vi "IandQ_Dat_ACQ.vi"() -> ()   [LabVIEW 2022 SP3]
doc: "I. Description:\nThis example demonstrates how to acquire a continuous amount of data (Waveform) using the DAQ device's internal clock.\n\nII. Instructions for Running:\n1. Create an analog input voltage channel.\n2. Set the rate for the sample clock. Additionally, define the sample mode to be continuous.\n3. Call the Start VI to start the acquisition.\n4. Read the waveform data in a loop until the user hits the stop button or an error occurs.\nNote: This example reads data from one or more channels and returns an array of data. Use the Index Array function to access an individual channel of data.\n5. Call the Clear Task VI to clear the Task.\n6. Use the popup dialog box to display an error if any.\n\nIV. I/O Connections Overview:\nMake sure your signal input terminal matches the Physical Channel I/O Control. For further connection information, refer to your hardware reference manual."
uses:
  <vilib>/Utility/error.llb/DialogType.ctl
  <vilib>/DAQmx/read.llb/DAQmx Read (Analog Wfm 1Chan NSamp).vi
  <vilib>/DAQmx/create/channels.llb/DAQmx Create Channel (AI-Voltage-Basic).vi
  <vilib>/DAQmx/configure/timing.llb/DAQmx Timing (Sample Clock).vi
  <vilib>/DAQmx/miscellaneous.llb/DAQmx Fill In Error Info.vi
panel:
  in  "Samples to Read":i32=1000
  in  "Physical Channel":tag="Dev1/ai0"
  in  "Minimum Value":dbl=-10.0 format="%0.2f"
  in  "Maximum Value":dbl=10.0 format="%0.2f"
  in  "stop":bool
  in  "Sample Rate":dbl=10000.0 caption="Sample Rate (Hz)" format="%0.2f"
  out "Measurement":waveform(dbl)(graph)
  # "For instructions, select Help>>Show Context Help"
  # "Channel Parameters"
  # "Timing Parameters"
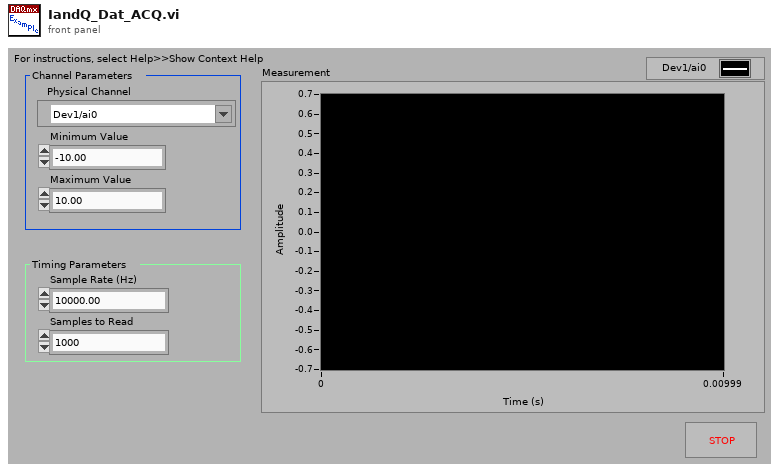
[diagram p1: front panel]
types:
  T1 = typedef "DialogType.ctl" = u16
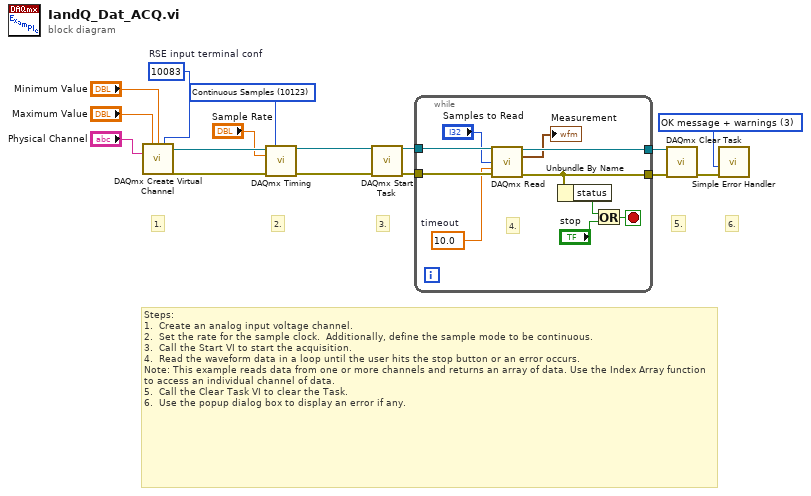
[diagram p0: block diagram]
diagram:
  w1 = 10083  # RSE input terminal conf
  w2 = T1 3 items=["no dialog", "OK message", "continue or stop message", "OK message + warnings", "continue/stop + warnings"] ("type of dialog (OK msg:1)")
  w7 = 10123 items=["Finite Samples"=10178, "Continuous Samples"=10123] ("sample mode")
  # "6."
  # "5."
  # "Steps: \n1.  Create an analog input voltage channel.\n2.  Set the rate for the sample clock.  Additionally, define the sample mode to be continuous.\n3.  Call the Start VI to start the acquisition.\n4.  Read the waveform data in a loop until the user hits the stop button or an error occurs.\nNote: This example reads data from one or more channels and returns an array of data. Use the Index Array function to access an individual channel of data.\n5.  Call the Clear Task VI to clear the Task.\n6.  Use the popup dialog box to display an error if any."
  # "3."
  # "2."
  # "1."
  n1 = call-poly <vilib>:"DAQmx Create Virtual Channel.vi"("maximum value"="Maximum Value", "minimum value"="Minimum Value", "input terminal configuration"=w1, "physical channels"="Physical Channel") -> ("task out"=w11:refnum<k21>, "error out"=w14:errorcluster)  [unwired: 5 in, 5 out]
  n2 = call-poly <vilib>:"DAQmx Timing.vi"("task/channels in"=w11, "sample mode"=w7, "rate"="Sample Rate", "error in"=w14) -> ("task out"=w6:refnum<k21>, "error out"=w5:errorcluster)  [unwired: 3 in, 7 out]
  n3 = call <vilib>:"DAQmx Start Task.vi"("task/channels in"=w6, "error in"=w5) -> ("task out"=w10:refnum<k21>, "error out"=w13:errorcluster)  [unwired: 12 out]
  n4 = while {
    tunnel: w13 -> [w26]
    tunnel: w10 -> [w25]
    tunnel: [w24] -> w9
    tunnel: [w22] -> w4
    stop <- w20 stop-if-true
    w18 = 10.0  # timeout
    # "4."
    n5 = call-poly <vilib>:"DAQmx Read.vi"("task/channels in"=w25, "number of samples per channel"="Samples to Read", "timeout"=w18, "error in"=w26) -> ("task out"=w24:refnum<k21>, "data"=→"Measurement":waveform(dbl), "error out"=w22:errorcluster)  [unwired: 9 out]
    n6 = Unbundle By Name(w22) -> ("status"=w21:bool)
    n7 = Or(x=w21, y="stop") -> (x .or. y?=w20:bool)
  }
  n8 = call <vilib>:"DAQmx Clear Task.vi"("task in"=w9, "error in"=w4) -> ("error out"=w12:errorcluster)  [unwired: 13 out]
  n9 = call <vilib>:"Simple Error Handler.vi"("type of dialog (OK msg:1)"=w2, "error in (no error)"=w12) -> ()  [unwired: 8 out]
